vi "Point getDistance.vi"(1 "point1":T1 {"y" format="%.2f"; "x" format="%.2f"}, 2 "point2":T1 {"y" format="%.2f"; "x" format="%.2f"}, 5 "error in (no error)":errorcluster) -> (15 "distance":dbl format="%.2f", 19 "error out":errorcluster)   [LabVIEW 2012]
doc: "contains"
uses:
  <resource>/Framework/Providers/Open_GDS/UML/General/Point/Point Point2D.ctl
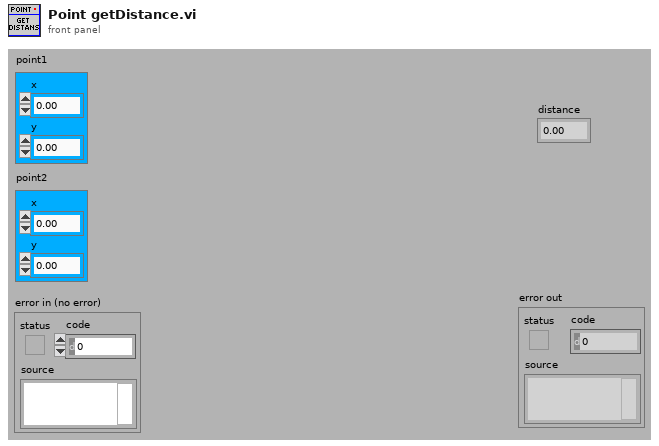
[diagram p1: front panel]
types:
  T1 = typedef "Point Point2D.ctl" = cluster{"x":dbl, "y":dbl}
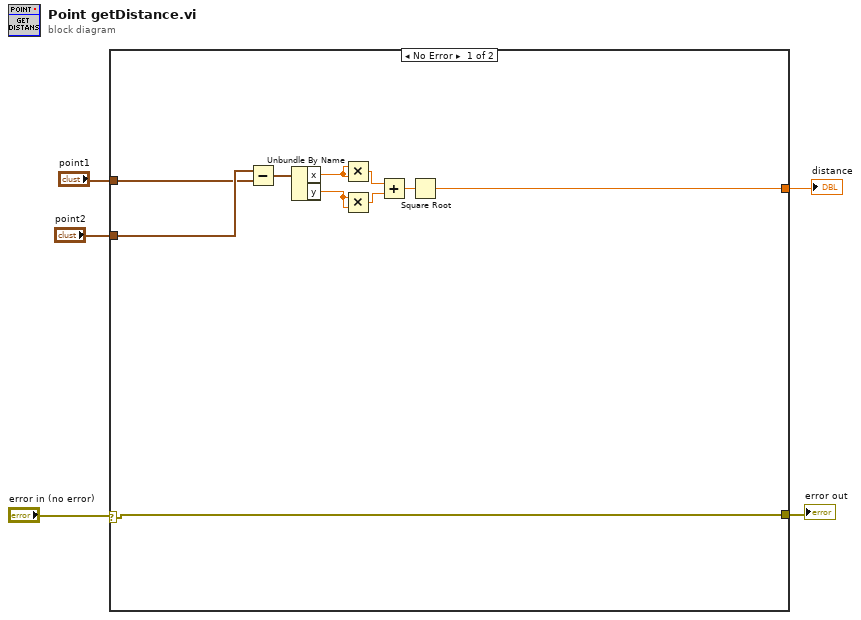
[diagram p0: block diagram]
diagram:
  n1 = case shown="No Error" "error in (no error)" {
    selector: "error in (no error)" -> [w15 w16]
    tunnel: [w15 w16] -> w5
    tunnel: "point1" -> [w13 _]
    tunnel: "point2" -> [w14 _]
    tunnel: [w6 _] -> w1
    frame No Error {
      n2 = Subtract(x=w14, y=w13) -> (x-y=w12:T1)
      n3 = Unbundle By Name(w12) -> ("x"=w10:dbl, "y"=w11:dbl)
      n4 = Multiply(x=w10, y=w10) -> (x*y=w8:dbl)
      n5 = Multiply(x=w11, y=w11) -> (x*y=w9:dbl)
      n6 = Add(x=w8, y=w9) -> (x+y=w7:dbl)
      n7 = Square Root(x=w7) -> (sqrt(x)=w6:dbl)
    }
    frame Error {
    }
  }
  "error out" <- w5
  "distance" <- w1
